vi "DrivePlanPath.vi"(1 "DrivePathPlanParams":T1={"max_velocity (in/s)"=100.0, "max_acceleration (in/s^2)"=80.0, "max_jerk (in/s^3)"=100.0, "dt(ms)"=40, "sample_count"=1000, "wheelbase_width (in)"=25.0} {"dt(ms)" items=["TrajectoryDuration_0ms"=0, "TrajectoryDuration_5ms"=5, "TrajectoryDuration_10ms"=10, "TrajectoryDuration_20ms"=20, "TrajectoryDuration_30ms"=30, "TrajectoryDuration_40ms"=40, "TrajectoryDuration_50ms"=50, "TrajectoryDuration_100ms"=100]}, 2 "DrivePlanRequest":T3) -> (0 "DrivePlanResponse":T6)   [LabVIEW 2017]
uses:
  PathPlannerSupport/TypeDefs/DrivePlanResponse.ctl
  Pathfinder/Pathfinder-LabVIEW/Pathfinder-Lib/VIs/Segment.ctl
  PathPlannerSupport/TypeDefs/DrivePlanRequest.ctl
  TypeDef/AutoWaypointType.ctl
  Pathfinder/Pathfinder-LabVIEW/Pathfinder-Lib/VIs/Waypoint.ctl
  PathPlannerSupport/TypeDefs/DrivePathfinderParams.ctl
  <vilib>/Rock Robotics/WPI/ThirdParty/Phoenix-LabVIEW/Motor Controller/Controls/CTRE_Phoenix_MotorControl_TrajectoryPointTimeDur.ctl
  Pathfinder/Pathfinder-LabVIEW/Pathfinder-Lib/Pathfinder.lvlib
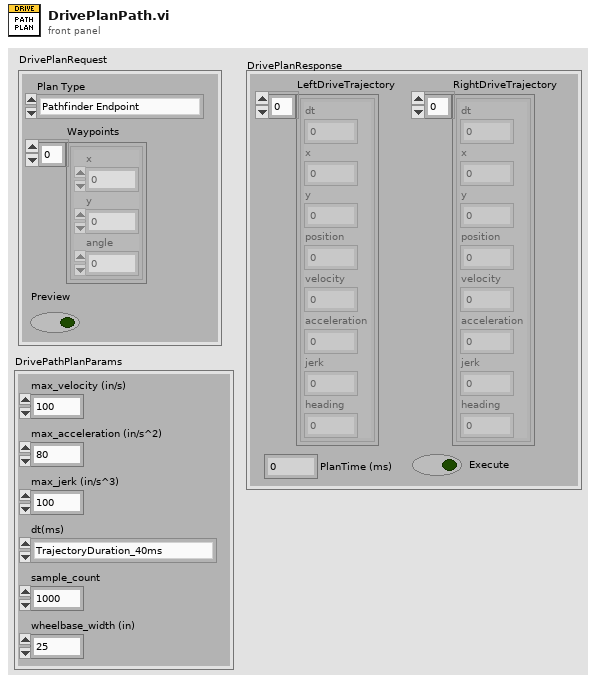
[diagram p1: front panel]
types:
  T1 = typedef "DrivePathfinderParams.ctl" = cluster{"max_velocity (in/s)":dbl, "max_acceleration (in/s^2)":dbl, "max_jerk (in/s^3)":dbl, "dt(ms)":T2, "sample_count":i32, "wheelbase_width (in)":dbl}
  T2 = typedef "CTRE_Phoenix_MotorControl_TrajectoryPointTimeDur.ctl" = i32
  T3 = typedef "DrivePlanRequest.ctl" = cluster{"Plan Type":T4, "Waypoints":T5[], "Preview":bool}
  T4 = typedef "AutoWaypointType.ctl" = enum16{"Pathfinder Endpoint", "Pathfinder Waypoint", "Zero-Radius Turn Endpoint", "Stationary", "Vision Assist Endpoint"}
  T5 = typedef "Pathfinder.lvlib/Waypoint.ctl" = cluster{"x":dbl, "y":dbl, "angle":dbl}
  T6 = typedef "DrivePlanResponse.ctl" = cluster{"LeftDriveTrajectory":T7[], "RightDriveTrajectory":T7[], "PlanTime (ms)":u32, "Execute":bool}
  T7 = typedef "Pathfinder.lvlib/Segment.ctl" = cluster{"dt":dbl, "x":dbl, "y":dbl, "position":dbl, "velocity":dbl, "acceleration":dbl, "jerk":dbl, "heading":dbl}
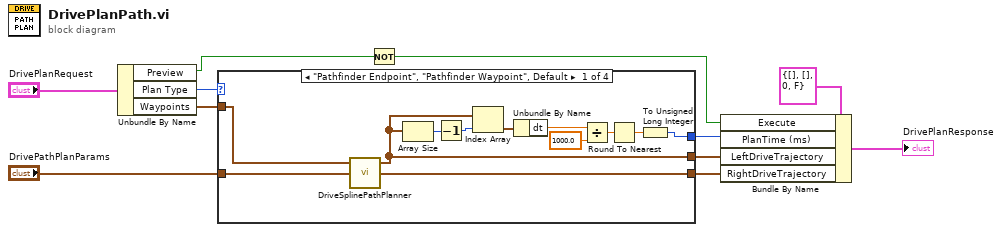
[diagram p0: block diagram]
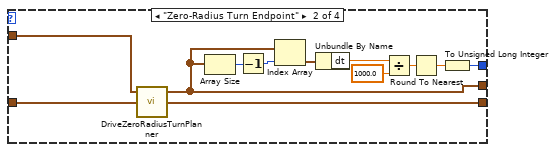
[diagram p2: hidden frame]
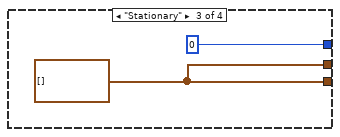
[diagram p3: hidden frame]
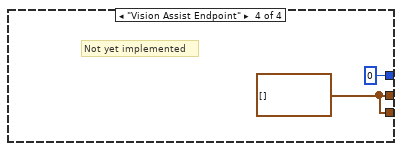
[diagram p4: hidden frame]
diagram:
  n1 = Unbundle By Name("DrivePlanRequest") -> ("Preview"=w6:bool, "Plan Type"=w11:T4, "Waypoints"=w1:T5[])
  n2 = case shown="\"Pathfinder Endpoint\", \"Pathfinder Waypoint\", Default" w11 {
    tunnel: "DrivePathPlanParams" -> [w23 w35 _ _]
    tunnel: [w20 w24 w37 w38] -> w4
    tunnel: [w22 w33 w37 w38] -> w3
    tunnel: [w13 w25 u32 0 ("PlanTime (ms)") u32 0 ("PlanTime (ms)")] -> w2
    tunnel: w1 -> [w12 w34 _ _]
    frame "Pathfinder Endpoint", "Pathfinder Waypoint", Default {
      n3 = call "DriveSplinePathPlanner.vi"("DrivePathPlanParams"=w23, "path"=w12) -> ("RightTrajectory"=w22:T7[], "LeftTrajectory"=w20:T7[])  [unwired: 1 in, 1 out]
      n4 = Array Size(array=w20) -> (size(s)=w21:i32)
      n5 = Decrement(x=w21) -> (x-1=w19:i32)
      n6 = Index Array(array=w20, index=w19) -> (element=w18:T7)
      n7 = Unbundle By Name(w18) -> ("dt"=w17:dbl)
      n8 = Divide(x=w17, y=1000.0) -> (x/y=w15:dbl)
      n9 = Round To Nearest(number=w15) -> (nearest integer value=w14:dbl)
      n10 = To Unsigned Long Integer(number=w14) -> (unsigned 32bit integer=w13:u32)
    }
    frame "Zero-Radius Turn Endpoint" {
      n11 = call "DriveZeroRadiusTurnPlanner.vi"("DrivePathPlanParams"=w35, "Waypoints"=w34) -> ("RightTrajectory"=w33:T7[], "LeftTrajectory"=w24:T7[])  [unwired: 2 in]
      n12 = Array Size(array=w24) -> (size(s)=w32:i32)
      n13 = Decrement(x=w32) -> (x-1=w31:i32)
      n14 = Index Array(array=w24, index=w31) -> (element=w30:T7)
      n15 = Unbundle By Name(w30) -> ("dt"=w29:dbl)
      n16 = Divide(x=w29, y=1000.0) -> (x/y=w27:dbl)
      n17 = Round To Nearest(number=w27) -> (nearest integer value=w26:dbl)
      n18 = To Unsigned Long Integer(number=w26) -> (unsigned 32bit integer=w25:u32)
    }
    frame "Stationary" {
      w37 = T7[] [] ("LeftTrajectory")
    }
    frame "Vision Assist Endpoint" {
      w38 = T7[] [] ("LeftTrajectory")
      # "Not yet implemented"
    }
  }
  n19 = Not(x=w6) -> (.not. x?=w5:bool)
  n20 = Bundle By Name(cluster=T6 {"LeftDriveTrajectory"=[], "RightDriveTrajectory"=[], "PlanTime (ms)"=0, "Execute"=FALSE} ("DrivePlanResponse"), "Execute"=w5, "PlanTime (ms)"=w2, "LeftDriveTrajectory"=w4, "RightDriveTrajectory"=w3) -> (→"DrivePlanResponse":T6)
